vi "Setup.vi"(8 "error in (no error)":errorcluster, 11 "Laser Diode Controller in":refnum<class "KLD101.lvclass">) -> (0 "error out":errorcluster, 3 "Laser Diode Controller out":refnum<class "KLD101.lvclass">)   [LabVIEW 2016, in "Laser Diode Controller.lvlib" / "KLD101.lvclass"]
uses:
  KLD101.lvclass
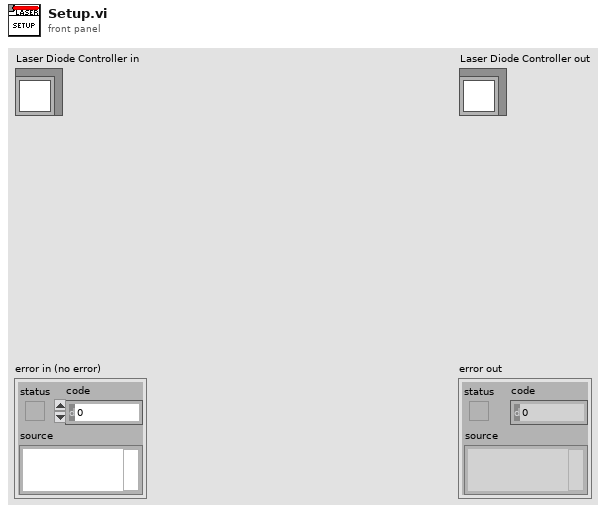
[diagram p1: front panel]
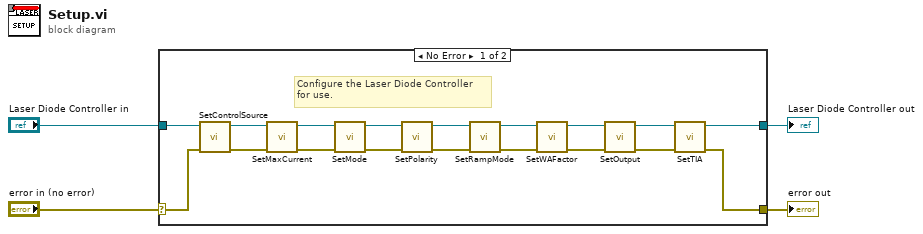
[diagram p0: block diagram]
diagram:
  n1 = case shown="No Error" "error in (no error)" {
    selector: "error in (no error)" -> [w19 w24]
    tunnel: [w5 w24] -> w3
    tunnel: [w7 w23] -> w1
    tunnel: "Laser Diode Controller in" -> [w20 w23]
    frame No Error {
      # "Configure the Laser Diode Controller\nfor use."
      n2 = call-dynamic "SetControlSource.vi"("error in (no error)"=w19, "Laser Diode Controller in"=w20) -> ("error out"=w13:errorcluster, "Laser Diode Controller out"=w14:refnum<class "KLD101.lvclass">)  [unwired: 8 in]
      n3 = call-dynamic "SetMaxCurrent.vi"("error in (no error)"=w13, "Laser Diode Controller in"=w14) -> ("error out"=w11:errorcluster, "Laser Diode Controller out"=w12:refnum<class "KLD101.lvclass">)  [unwired: 8 in]
      n4 = call-dynamic "SetMode.vi"("error in (no error)"=w11, "Laser Diode Controller in"=w12) -> ("error out"=w21:errorcluster, "Laser Diode Controller out"=w22:refnum<class "KLD101.lvclass">)  [unwired: 8 in]
      n5 = call-dynamic "SetPolarity.vi"("error in (no error)"=w21, "Laser Diode Controller in"=w22) -> ("error out"=w9:errorcluster, "Laser Diode Controller out"=w10:refnum<class "KLD101.lvclass">)  [unwired: 8 in]
      n6 = call-dynamic "SetRampMode.vi"("error in (no error)"=w9, "Laser Diode Controller in"=w10) -> ("error out"=w16:errorcluster, "Laser Diode Controller out"=w18:refnum<class "KLD101.lvclass">)  [unwired: 8 in]
      n7 = call-dynamic "SetWAFactor.vi"("error in (no error)"=w16, "Laser Diode Controller in"=w18) -> ("error out"=w15:errorcluster, "Laser Diode Controller out"=w17:refnum<class "KLD101.lvclass">)  [unwired: 8 in]
      n8 = call-dynamic "SetOutput.vi"("error in (no error)"=w15, "Laser Diode Controller in"=w17) -> ("error out"=w6:errorcluster, "Laser Diode Controller out"=w8:refnum<class "KLD101.lvclass">)  [unwired: 8 in]
      n9 = call-dynamic "SetTIA.vi"("error in (no error)"=w6, "Laser Diode Controller in"=w8) -> ("error out"=w5:errorcluster, "Laser Diode Controller out"=w7:refnum<class "KLD101.lvclass">)  [unwired: 8 in]
    }
    frame Error {
    }
  }
  "error out" <- w3
  "Laser Diode Controller out" <- w1
